vi "excelExport.vi"(8 "error in (no error)":errorcluster, 11 "SR430Class.lvclass (in)":refnum<class "SR430Class.lvclass">) -> (0 "error out":errorcluster, 3 "SR430Class.lvclass (out)":refnum<class "SR430Class.lvclass">)   [LabVIEW 2015, in "SR430Class.lvclass"]
uses:
  class/SR430Class.lvclass
  class/SR430Class.lvclass/SR430Class.ctl
  support/SR430 Driver/SR430Driver.lvlib
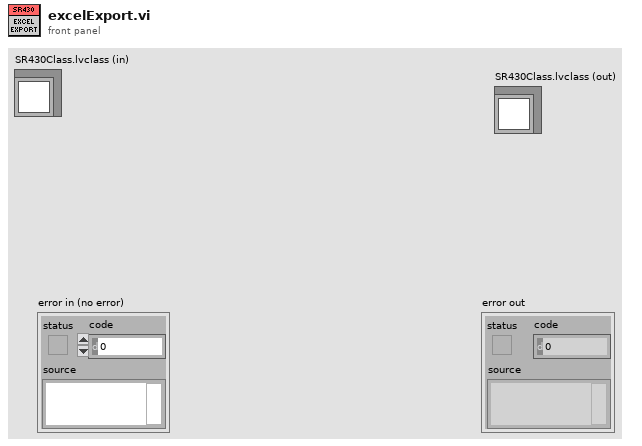
[diagram p1: front panel]
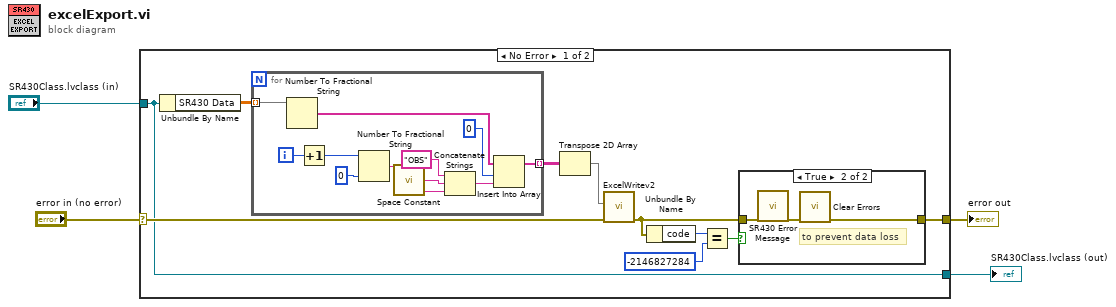
[diagram p0: block diagram]
diagram:
  n1 = case shown="No Error" "error in (no error)" {
    selector: "error in (no error)" -> [w8 w31]
    tunnel: [w7 w31] -> w3
    tunnel: [w6 w30] -> w2
    tunnel: "SR430Class.lvclass (in)" -> [w6 w30]
    frame No Error {
      n2 = Unbundle By Name(w6) -> ("SR430 Data"=w5:dbl[][])
      n3 = for {
        tunnel: w5 -> [w23] mode=indexing
        tunnel: [w20] -> w13 mode=indexing
        i -> [w25]
        n4 = Number To Fractional String(number=w23) -> (F-format string=w22:string[])  [unwired: 3 in]
        n5 = Increment(x=w25) -> (x+1=w26:i32)
        n6 = Number To Fractional String(number=w26, precision (6)=i16 0) -> (F-format string=w29:string)  [unwired: 2 in]
        n7 = call <vilib>:"Space Constant.vi"() -> ("String"=w27:string)
        n8 = Concatenate Strings("OBS" ("string"), w27, w29) -> (w21:string)
        n9 = Insert Into Array(array=w22, index=0, new element=w21) -> (w20:string[])
      }
      n10 = Transpose 2D Array(2D array=w13) -> (transposed array=w14:string[][])
      n11 = call "ExcelWritev2.vi"("error in"=w8, "Data"=w14) -> ("error out"=w9:errorcluster)  [unwired: 9 in]
      n12 = Unbundle By Name(w9) -> ("code"=w11:i32)
      n13 = Equal?(x=w11, y=-2146827284) -> (x = y?=w10:bool)
      n14 = case shown="True" w10 {
        tunnel: w9 -> [w15 w17]
        tunnel: [w15 w18] -> w7
        frame False {
        }
        frame True {
          # "to prevent data loss"
          n15 = call "SR430 Error Message.vi"("error in (no error)"=w17) -> ("error out"=w16:errorcluster)  [unwired: 15 in, 3 out]
          n16 = call <vilib>:"Clear Errors.vi"("error in (no error)"=w16) -> ("error out"=w18:errorcluster)  [unwired: 5 in, 1 out]
        }
      }
    }
    frame Error {
    }
  }
  "error out" <- w3
  "SR430Class.lvclass (out)" <- w2
